vi "torque_and_rpm_average.vi"(6 "mean 2":dbl, 9 "rpm_offszet":dbl, 10 "tq_offszet":dbl, 11 "mean":dbl) -> (1 "Numeric 2":dbl, 2 "Numeric 3":dbl, 3 "Numeric 4":dbl, 4 "Numeric":dbl)   [LabVIEW 2014]
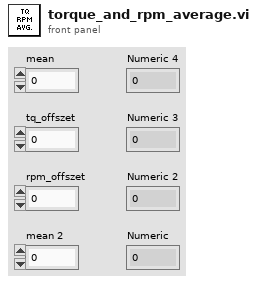
[diagram p1: front panel]
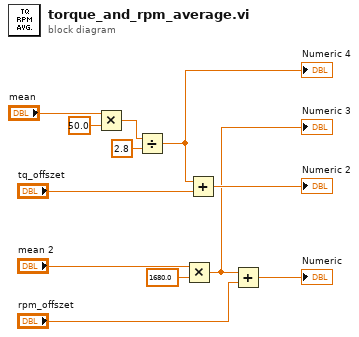
[diagram p0: block diagram]
diagram:
  n1 = Multiply(x="mean", y=50.0) -> (x*y=w6:dbl)
  n2 = Divide(x=w6, y=2.8) -> (x/y=w7:dbl)
  "Numeric 4" <- w7
  n3 = Multiply(x="mean 2", y=1680.0) -> (x*y=w8:dbl)
  "Numeric 3" <- w8
  n4 = Add(x=w7, y="tq_offszet") -> (x+y=→"Numeric 2":dbl)
  n5 = Add(x=w8, y="rpm_offszet") -> (x+y=→"Numeric":dbl)
